vi "Init.vi"(8 "error in (no error)":errorcluster, 9 "Intrs Configs":T2, 10 "Excitation":T1, 11 "ILock-In Remote Actor in":refnum<class "ILock-In Remote Actor.lvclass">) -> (0 "error out":errorcluster, 3 "ILock-In Remote Actor out":refnum<class "ILock-In Remote Actor.lvclass">)   [LabVIEW 2023, in "Lock-In Remote Actor - Interface.lvlib" / "ILock-In Remote Actor.lvclass"]
uses:
  ILock-In Remote Actor.lvclass
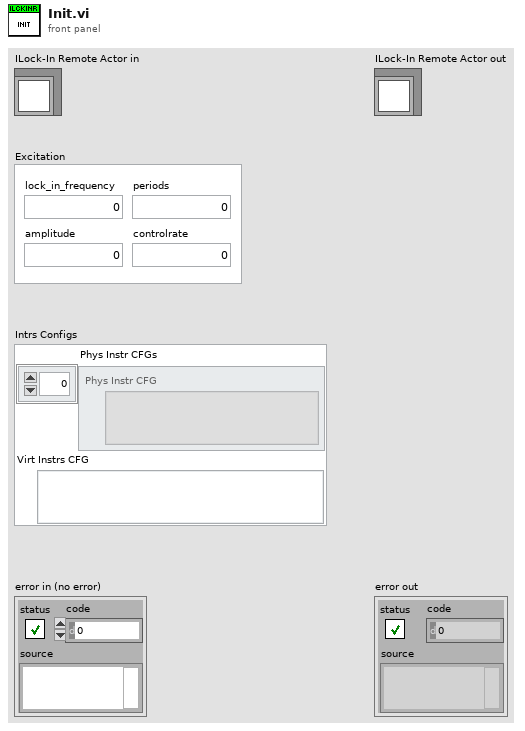
[diagram p1: front panel]
types:
  T1 = cluster{"lock_in_frequency":dbl, "amplitude":dbl, "periods":dbl, "controlrate":dbl}
  T2 = cluster{"Phys Instr CFGs":path[], "Virt Instrs CFG":path}
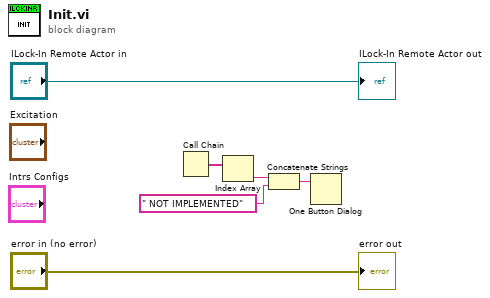
[diagram p0: block diagram]
diagram:
  n1 = Call Chain() -> (call chain=w4:string[])
  n2 = Index Array(array=w4) -> (element=w2:string)  [unwired: 1 in]
  n3 = Concatenate Strings(w2, " NOT IMPLEMENTED" ("string")) -> (w3:string)
  n4 = One Button Dialog(message=w3) -> ()  [unwired: 1 in, 1 out]
  "error out" <- "error in (no error)"
  "ILock-In Remote Actor out" <- "ILock-In Remote Actor in"
